vi "Read Format String.vi"(9 "NumericText in":refnum<class "Digital.lvclass">) -> (3 "NumericText out":refnum<class "Digital.lvclass">, 4 "Format String":string)   [LabVIEW 2014, in "Raspberry Pi Compatible Compiler for LabVIEW.lvlib" / "Digital.lvclass"]
uses:
  Digital.lvclass
  Digital.lvclass/Digital.ctl
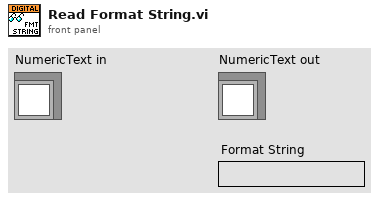
[diagram p1: front panel]
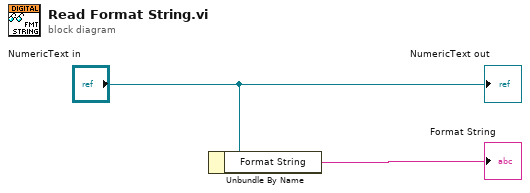
[diagram p0: block diagram]
diagram:
  n1 = Unbundle By Name("NumericText in") -> ("Format String"=→"Format String":string)
  "NumericText out" <- "NumericText in"
